vi "StoreImageFromString.vi"(0 "reference in":refnum<class "LcPictureBox.lvclass">, 1 "ImageName":string, 2 "ImageNames":string[](array[string]), 3 "ImageFileContent":string, 5 "error in (no error)":errorcluster) -> (14 "reference out":refnum<class "LcPictureBox.lvclass">, 19 "error out":errorcluster)   [LabVIEW 2020, in "LcPictureBox.lvclass"]
uses:
  LcPictureBox.lvclass
  <vilib>/Utility/miscctls.llb/LVMapReplaceAction.ctl
  System.Drawing
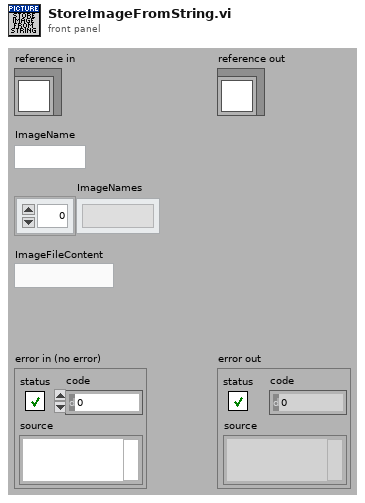
[diagram p1: front panel]
types:
  T1 = typedef "LVMapReplaceAction.ctl" = enum32{"Modify Entry only if found", "Add or Modify Entry", "Delete Entry"}
  T2 = cluster{"ImageOut":refnum<k24>, "ImageSize":cluster{"Width":i32, "Height":i32}}
  T3 = typedef "LcPictureBox.lvclass/ObjectAttributes.ctl" = cluster{"PictureBox":refnum<k24>, "ImageSize":cluster{"Width":i32, "Height":i32}, "PenMemory":map{cluster{"Alpha(100%)":dbl, "Color(Black)":u32, "Pen(Width=1, Solid)":T4}, refnum<k24>}, "GraphicsRef":refnum<k24>, "BrushMemory":map{cluster{"Alpha(100%)":dbl, "Color(Black)":u32}, refnum<k24>}, "Images":refnum<k24>[], "ImageIndex":i32, "BgColor(None)":u32, "LoadedImages":map{string, cluster{"ImageOut":refnum<k24>, "ImageSize":cluster{"Width":i32, "Height":i32}}}, "ColorsMemory":map{cluster{"Alpha(100%)":dbl, "Color(Black)":u32}, refnum<k24>}, "CacheSize":i32, "PictureBoxActiveXReference":refnum<vi>, "Scale":sgl, "Offset":cluster{"x":sgl, "y":sgl}, "zoom_center":cluster{"X":i32, "Y":i32}, "ImagesCreated":refnum<k24>[]}
  T4 = typedef "LcPictureBox.lvclass/Pen.ctl" = cluster{"Width":u16, "Style":enum32{"Solid", "Dash", "Dot", "DashDot", "DashDotDot"}}
  T5 = map{string, cluster{"ImageOut":refnum<k24>, "ImageSize":cluster{"Width":i32, "Height":i32}}}
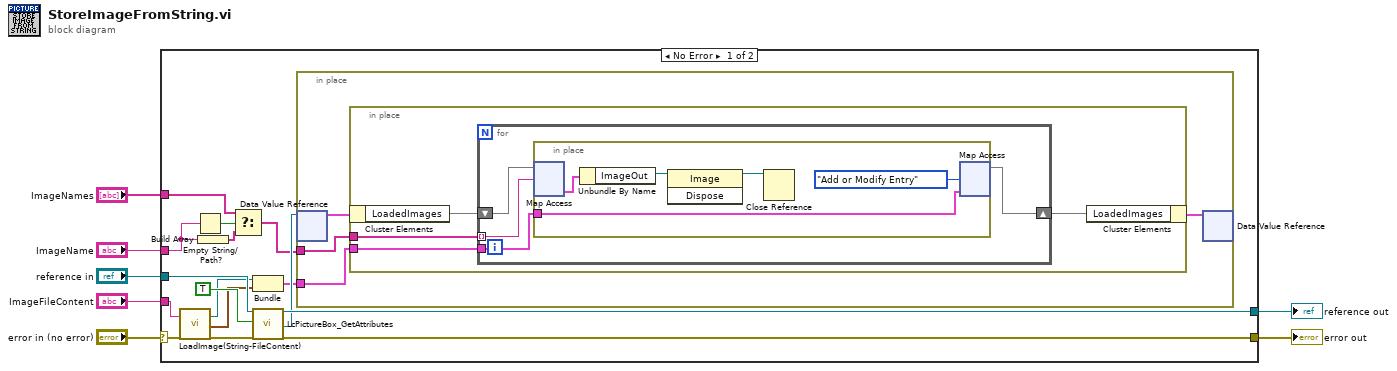
[diagram p0: block diagram]
diagram:
  n1 = case shown="No Error" "error in (no error)" {
    selector: "error in (no error)" -> [w20 w42]
    tunnel: [w14 w42] -> w6
    tunnel: [w22 w41] -> w4
    tunnel: "reference in" -> [w23 w41]
    tunnel: "ImageFileContent" -> [w8 _]
    tunnel: "ImageName" -> [w9 _]
    tunnel: "ImageNames" -> [w12 _]
    frame No Error {
      n2 = call "LoadImage(String-FileContent).vi"("ImageFileContent"=w8, "error in (no error)"=w20) -> ("ImageOut"=w17:refnum<k24>, "ImageSize"=w16:cluster{"Width":i32, "Height":i32}, "error out"=w18:errorcluster)  [unwired: 15 in]
      n3 = Empty String/Path?(string/path=w9) -> (empty?=w13:bool)
      n4 = Build Array(w9) -> (w11:string[])
      n5 = Select(t=w12, s=w13, f=w11) -> (s? t:f=w10:string[])
      n6 = Bundle("ImageOut"=w17, "ImageSize"=w16) -> (w15:T2)  [unwired: 1 in]
      n7 = call "LcPictureBox_GetAttributes.vi"("reference in"=w23, "OnlyGetDvrReference(False)"=TRUE, "error in (no error)"=w18) -> ("reference out"=w22:refnum<class "LcPictureBox.lvclass">, "DataRef"=w19:refnum<data-value>, "error out"=w14:errorcluster)  [unwired: 13 in, 1 out]
      n8 = in-place {
        in-place-border: w15 -> [w25]
        in-place-border: w10 -> [w24]
        n9 = in-place-dvr #1(w19) -> (w27:T3)  [unwired: 1 out]
        n10 = in-place {
          in-place-border: w25 -> [w29]
          in-place-border: w24 -> [w28]
          n11 = in-place-cluster #2(w27) -> ("LoadedImages"=w31:T5)
          n12 = for {
            tunnel: w29 -> [w33]
            tunnel: w28 -> [w32] mode=indexing
            shift-right: [w34] -> w30
            shift-left: w31 -> [w35]
            n13 = in-place {
              in-place-border: w33 -> [w39]
              n14 = in-place-map #3(w35, w32) -> (w38:T2)  [unwired: 1 in, 1 out]
              n15 = Unbundle By Name(w38) -> ("ImageOut"=w37:refnum<k24>)
              n16 = invoke class="Image" method="Dispose"(reference=w37) -> (reference out=w36:refnum<k24>)  [unwired: 2 in, 2 out]
              n17 = Close Reference(reference=w36) -> ()  [unwired: 1 in, 1 out]
              n18 = in-place-map #3(w39, LVMapReplaceAction."Add or Modify Entry" ("action")) -> (w34:T5)  [unwired: 2 out]
            }
          }
          n19 = in-place-cluster #2("LoadedImages"=w30) -> (w26:T3)
        }
        n20 = in-place-dvr #1(w26) -> ()  [unwired: 2 out]
      }
    }
    frame Error {
    }
  }
  "error out" <- w6
  "reference out" <- w4
